vi "GetCameraStatus.vi"(0 "TCP/IP ID":refnum<k5>, 2 "error in (no error)":errorcluster) -> (3 "CCD temp":string, 4 "Backplate Temp":string, 5 "Vacuum Pressure":string, 6 "error out":errorcluster)   [LabVIEW 2015]
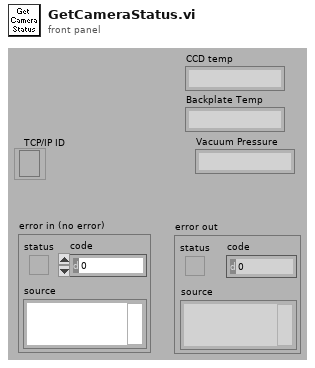
[diagram p1: front panel]
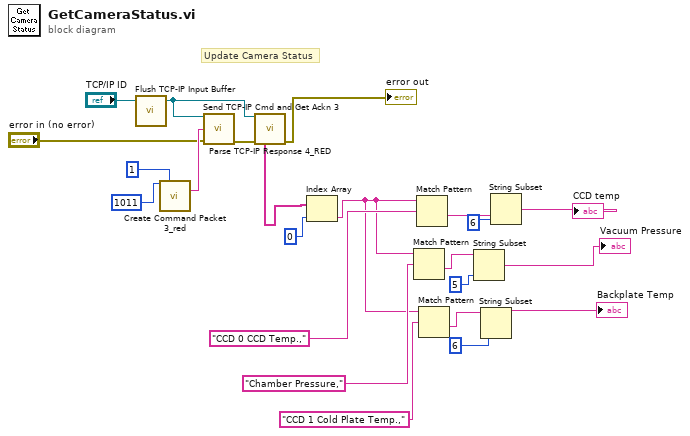
[diagram p0: block diagram]
diagram:
  # "Update Camera Status"
  n1 = call "Flush TCP-IP Input Buffer.vi"("TCP/IP ID"="TCP/IP ID") -> ("TCP/IP ID Out"=w19:refnum<k5>)  [unwired: 4 in]
  n2 = call "Create Command Packet 3_red.vi"("Function #"=u16 1011, "Camera ID (1)"=u16 1 ("Function #")) -> ("Cmd Packet"=w23:string)  [unwired: 13 in]
  n3 = call "Send TCP-IP Cmd and Get Ackn 3.vi"("TCP/IP ID In"=w19, "Cmd Packet"=w23, "error in (no error)"="error in (no error)") -> ("error out"=w20:errorcluster)  [unwired: 6 in, 6 out]
  n4 = call "Parse TCP-IP Response 4_RED.vi"("TCP/IP ID"=w19, "error in (no error)"=w20) -> ("Status Array"=w12:string[], "error out"=→"error out":errorcluster)  [unwired: 3 in, 9 out]
  n5 = Index Array(array=w12, index=0) -> (element=w2:string)
  n6 = Match Pattern(string=w2, regular expression="Chamber Pressure,") -> (after substring=w7:string)  [unwired: 1 in, 3 out]
  n7 = Match Pattern(string=w2, regular expression="CCD 0 CCD Temp.,") -> (after substring=w1:string)  [unwired: 1 in, 3 out]
  n8 = Match Pattern(string=w2, regular expression="CCD 1 Cold Plate Temp.,") -> (after substring=w8:string)  [unwired: 1 in, 3 out]
  n9 = String Subset(string=w7, length (rest)=5) -> (substring=→"Vacuum Pressure":string)  [unwired: 1 in]
  n10 = String Subset(string=w8, length (rest)=6) -> (substring=→"Backplate Temp":string)  [unwired: 1 in]
  n11 = String Subset(string=w1, length (rest)=6) -> (substring=→"CCD temp":string)  [unwired: 1 in]
